vi "Rinocloud_HTTP_children.vi"(3 "error in (no error)":errorcluster, 5 "id":string) -> (0 "error out":errorcluster, 1 "Status":T2={"headers"="", "body"="", "ID"="", "Saved"=TRUE}, 2 "metadata array":T1(array[cluster]))   [LabVIEW 2013, in "Rinocloud Library.lvlib"]
uses:
  Rinocloud Library.lvlib
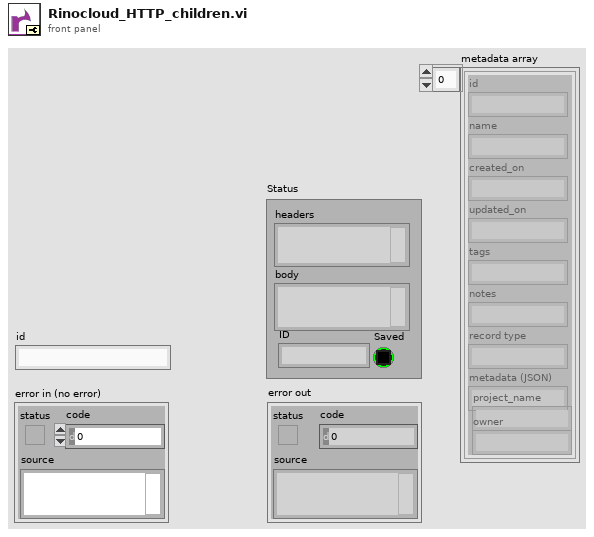
[diagram p1: front panel]
types:
  T1 = cluster{"id":string, "name":string, "created_on":string, "updated_on":string, "tags":string, "notes":string, "record type":string, "metadata (JSON)":string, "project_name":string, "owner":string}[]
  T2 = cluster{"headers":string, "body":string, "ID":string, "Saved":bool}
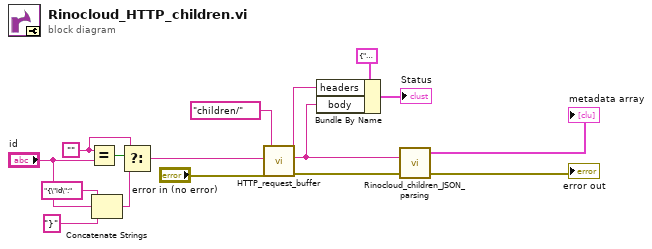
[diagram p0: block diagram]
diagram:
  w16 = ""
  n1 = Equal?(x=w16, y="id") -> (x = y?=w12:bool)
  n2 = Concatenate Strings("{\"id\":" ("string"), "id", "}" ("string")) -> (w14:string)
  n3 = Select(t=w16, s=w12, f=w14) -> (s? t:f=w13:string)
  n4 = call "HTTP_request_buffer.vi"("error in (no error)"="error in (no error)", "JSON payload"=w13, "Endpoint"="children/") -> ("error out"=w9:errorcluster, "body"=w10:string, "headers"=w8:string)  [unwired: 2 in]
  n5 = Bundle By Name(cluster=T2 {"headers"="", "body"="", "ID"="", "Saved"=TRUE} ("Status 2"), "headers"=w8, "body"=w10) -> (→"Status":T2)
  n6 = call "Rinocloud_children_JSON_parsing.vi"("error in (no error)"=w9, "JSON string"=w10) -> ("error out"=→"error out":errorcluster, "metadata array"=→"metadata array":T1)  [unwired: 2 in]
